vi "ABC Find Open.vi"(4 "UART":refnum<vi>, 5 "ComPort":refnum<visa-resource-name>, 6 "Data":refnum<vi>, 7 "DaqTask":refnum<k21>, 8 "ErrIn":errorcluster, 9 "#Step":i32, 10 "Dir":T1, 11 "DataIn":dbl[](array[numeric])=[0.0]) -> (0 "ErrOut":errorcluster, 1 "FrontOpen":dbl, 2 "BackOpen":dbl, 3 "DataOut":dbl[](array[numeric]))   [LabVIEW 2020]
uses:
  <userlib>/Amira UART/Public/TypeDefs/AUART StepDir.ctl
  <vilib>/DAQmx/read.llb/DAQmx Read (Digital 1D Bool 1Chan 1Samp).vi
  <vilib>/DAQmx/miscellaneous.llb/DAQmx Fill In Error Info.vi
  <userlib>/Amira UART/Amira UART.lvclass
  <userlib>/KQD LabVIEW User/Serial/Serial.lvlib
panel:
  out "FrontSW":bool
  out "BackSW":bool
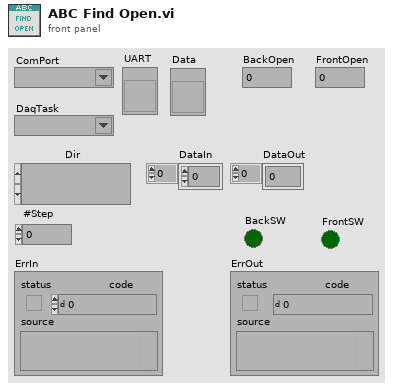
[diagram p1: front panel]
types:
  T1 = typedef "Amira UART.lvclass/AUART StepDir.ctl" = enum16{"", "compress", "decompress"}
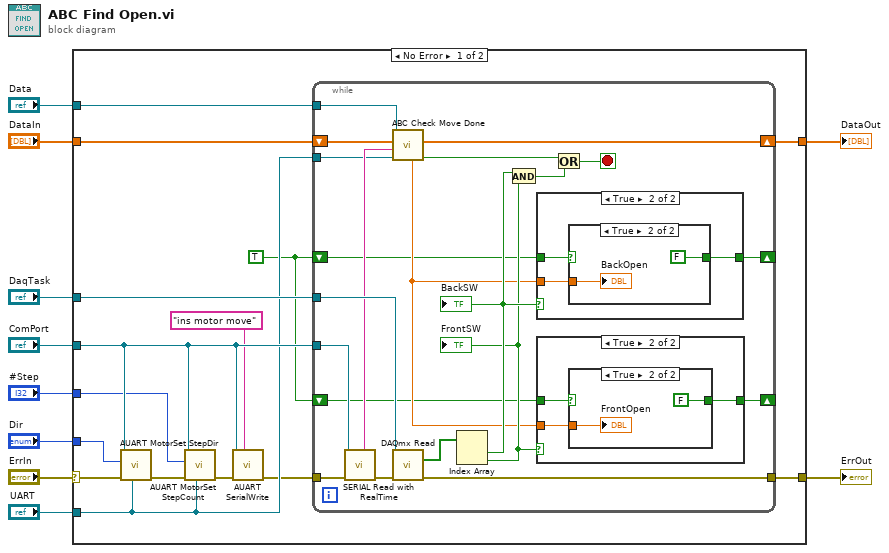
[diagram p0: block diagram]
diagram:
  n1 = case shown="No Error" "ErrIn" {
    selector: "ErrIn" -> [w19 w61]
    tunnel: "UART" -> [w18 _]
    tunnel: "DaqTask" -> [w25 _]
    tunnel: [w24 w61] -> w8
    tunnel: "DataIn" -> [w23 w62]
    tunnel: [w22 w62] -> w6
    tunnel: "ComPort" -> [w20 _]
    tunnel: "Data" -> [w17 _]
    tunnel: "Dir" -> [w13 _]
    tunnel: "#Step" -> [w12 _]
    frame No Error {
      w11 = TRUE
      n2 = call <userlib>:"AUART MotorSet StepDir.vi"("UART"=w18, "ErrIn"=w19, "step_dir"=w13, "Port"=w20) -> ("ErrOut"=w21:errorcluster)  [unwired: 7 in]
      n3 = call <userlib>:"AUART MotorSet StepCount.vi"("UART"=w18, "ErrIn"=w21, "step_count"=w12, "Port"=w20) -> ("ErrOut"=w16:errorcluster)  [unwired: 7 in]
      n4 = call <userlib>:"AUART SerialWrite.vi"("Cmd"="ins motor move", "ErrIn"=w16, "Port"=w20) -> ("ErrOut"=w15:errorcluster)  [unwired: 7 in, 1 out]
      n5 = while {
        tunnel: w25 -> [w45]
        tunnel: w17 -> [w39]
        tunnel: w20 -> [w44]
        shift-right: [w36] -> w22
        shift-left: w23 -> [w40]
        tunnel: w15 -> [w43]
        tunnel: [w41] -> w24
        tunnel: w18 -> [w37]
        shift-right: [w28] -> _
        shift-left: w11 -> [w29]
        shift-right: [w26] -> _
        shift-left: w11 -> [w27]
        stop <- w32 stop-if-true
        n6 = call <userlib>:"SERIAL Read with RealTime.vi"("ErrIn"=w43, "PortIn"=w44) -> ("ErrOut"=w42:errorcluster, "Response"=w38:string)  [unwired: 7 in, 1 out]
        n7 = call "ABC Check Move Done.vi"("UART"=w37, "Response"=w38, "DataIn"=w40, "Data"=w39) -> ("Done"=w31:bool, "DataOut"=w36:dbl[], "Position"=w33:dbl)  [unwired: 5 in]
        n8 = call-poly <vilib>:"DAQmx Read.vi"("task/channels in"=w45, "error in"=w42) -> ("data"=w46:bool[], "error out"=w41:errorcluster)  [unwired: 11 in, 1 out]
        n9 = Index Array(array=w46) -> (element #1=w35:bool, element #2=w34:bool)  [unwired: 2 in]
        "BackSW" <- w35
        "FrontSW" <- w34
        n10 = And(x=w35, y=w34) -> (x .and. y?=w30:bool)
        n11 = case shown="True" w35 {
          tunnel: w33 -> [_ w57]
          tunnel: w29 -> [w54 w56]
          tunnel: [w54 w55] -> w28
          frame False {
          }
          frame True {
            n12 = case shown="True" w56 {
              selector: w56 -> [w58 _]
              tunnel: w57 -> [_ w60]
              tunnel: [w58 FALSE] -> w55
              frame False {
              }
              frame True {
                "BackOpen" <- w60
              }
            }
          }
        }
        n13 = case shown="True" w34 {
          tunnel: w33 -> [_ w50]
          tunnel: w27 -> [w47 w49]
          tunnel: [w47 w48] -> w26
          frame False {
          }
          frame True {
            n14 = case shown="True" w49 {
              selector: w49 -> [w51 _]
              tunnel: w50 -> [_ w53]
              tunnel: [w51 FALSE] -> w48
              frame False {
              }
              frame True {
                "FrontOpen" <- w53
              }
            }
          }
        }
        n15 = Or(x=w31, y=w30) -> (x .or. y?=w32:bool)
      }
    }
    frame Error {
    }
  }
  "ErrOut" <- w8
  "DataOut" <- w6
